vi "Add To Queue.vi"(8 "error in":errorcluster, 9 "Data":variant, 10 "Priority":i32=1, 11 "Action":T1) -> (0 "error out":errorcluster)   [LabVIEW 2015]
uses:
  Sprocket/src/Action/Action Name.ctl
  Sprocket/src/Refname/Queues.ctl
  Sprocket/src/Refname/Refname to String (Queue).vi
  Sprocket/lib/Sprocket.lvlib
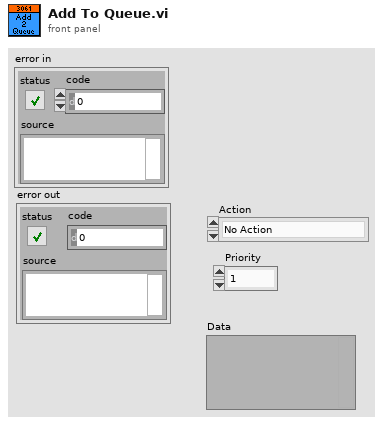
[diagram p1: front panel]
types:
  T1 = typedef "Sprocket.lvlib/Action Name.ctl" = enum16{"No Action", "Drive Train Left", "Drive Train Right", "Drive Train Both", "Collector Motor Eject", "Collector Motor Collect", "Collector Motor Stop", "Collector Extend", "Collector Retract", "Shifter High", "Shifter Low"}
  T2 = typedef "Sprocket.lvlib/Queues.ctl" = enum16{"Input", "Drive", "Collector", "Shifter"}
  T3 = cluster{"Action":T1, "Priority":i32, "Data":variant}
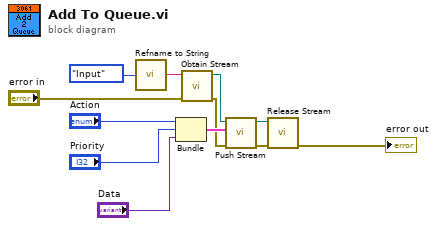
[diagram p0: block diagram]
diagram:
  n1 = call-poly "Refname to String.vi"("Queue Refname"=Queues."Input" ("Refname (Queue)")) -> ("Refnum Name"=w10:string)
  n2 = Bundle("Action"="Action", "Priority"="Priority", "Data"="Data") -> (w4:T3)  [unwired: 1 in]
  n3 = call "Obtain Stream.vi"("error in (no error)"="error in", "Name"=w10) -> ("error out"=w2:errorcluster, "stream out"=w7:refnum<queue>)  [unwired: 8 in]
  n4 = call "Push Stream.vi"("error in (no error)"=w2, "action"=w4, "stream in"=w7) -> ("error out"=w9:errorcluster, "stream out"=w6:refnum<queue>)  [unwired: 7 in]
  n5 = call "Release Stream.vi"("error in (no error)"=w9, "stream in"=w6) -> ("error out"=→"error out":errorcluster)  [unwired: 8 in, 1 out]
